vi "ShooterSpeedChoose.vi"(7 "Shooter OFF":bool, 9 "Close 3pt Shot Button":bool, 10 "Far 3pt Shot Button":bool, 11 "Feedershot Button":bool) -> (3 "Shooter Speed":T1(ring))   [LabVIEW 2012]
uses:
  Robot Global Data.vi
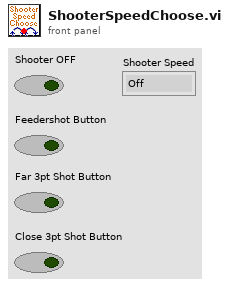
[diagram p1: front panel]
types:
  T1 = enum16{"Off", "Close Pyramid 3pt", "Far Pyramid 3pt", "Feeder Shot"}
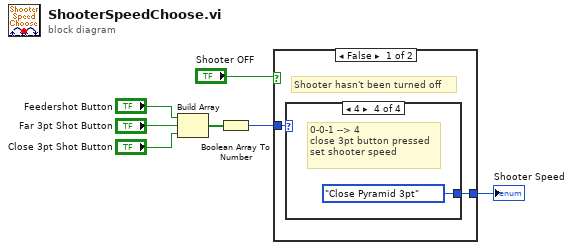
[diagram p0: block diagram]
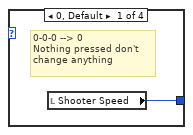
[diagram p2: hidden frame]
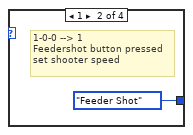
[diagram p3: hidden frame]
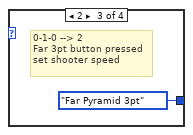
[diagram p4: hidden frame]
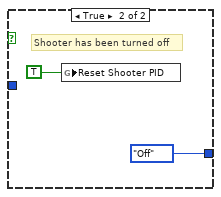
[diagram p5: hidden frame]
diagram:
  n1 = Build Array("Feedershot Button", "Far 3pt Shot Button", "Close 3pt Shot Button") -> (w7:bool[])
  n2 = Boolean Array To Number(Boolean array=w7) -> (number=w5:u32)
  n3 = case shown="False" "Shooter OFF" {
    tunnel: w5 -> [w9 _]
    tunnel: [w8 T1."Off" ("Shooter Speed")] -> w1
    frame False {
      # "Shooter hasn't been turned off"
      n4 = case shown="4" w9 {
        tunnel: [w10 T1."Feeder Shot" ("Shooter Speed") T1."Far Pyramid 3pt" ("Shooter Speed") T1."Close Pyramid 3pt" ("Shooter Speed")] -> w8
        frame 0, Default {
          # "0-0-0 --> 0\nNothing pressed don't \nchange anything"
          n5 = local read "Shooter Speed"() -> (w10:T1)
        }
        frame 1 {
          # "1-0-0 --> 1\nFeedershot button pressed\nset shooter speed"
        }
        frame 2 {
          # "0-1-0 --> 2\nFar 3pt button pressed\nset shooter speed"
        }
        frame 4 {
          # "0-0-1 --> 4\nclose 3pt button pressed\nset shooter speed"
        }
      }
    }
    frame True {
      # "Shooter has been turned off"
      n6 = global write "Robot Global Data.vi" "Reset Shooter PID"(TRUE) -> ()
    }
  }
  "Shooter Speed" <- w1
